vi "权值计算.vi"(0 "当前棋盘状态":i32[][](array[numeric])) -> (3 "权值最大的三个位置":dbl[][](array[numeric]), 4 "当前棋盘状态":i32[][](array[numeric]), 8 "行":sgl, 10 "列":i16, 13 "黑子最大权值":sgl, 14 "白子最大权值":sgl format="%#_0f", 15 "白子权值大于黑子？":bool)   [LabVIEW 2018]
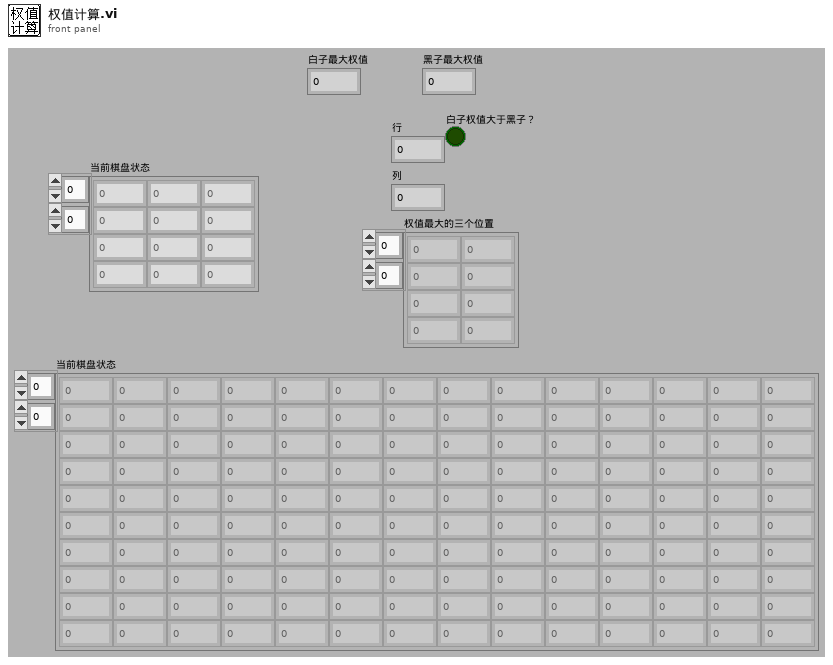
[diagram p1: front panel]
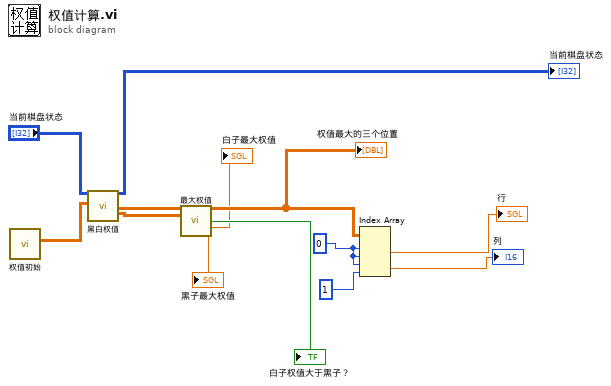
[diagram p0: block diagram]
diagram:
  w7 = 0 ("index (row)")
  n1 = call "权值初始.vi"() -> ("初始棋盘权值"=w12:sgl[][])  [unwired: 11 in]
  n2 = call "黑白权值.vi"("输入棋盘状态"="当前棋盘状态", "初始棋盘权值"=w12) -> ("输出棋盘状态"=→"当前棋盘状态":i32[][], "白子棋盘总权值"=w10:sgl[][], "黑子棋盘总权值"=w9:sgl[][])  [unwired: 15 in]
  n3 = call "最大权值.vi"("白子棋盘权值"=w10, "黑子棋盘权值"=w9) -> ("权值最大的前三个位置"=w8:dbl[][], "白子权值勤大于黑子？"=→"白子权值大于黑子？":bool, "白子最大权值"=→"白子最大权值":sgl, "黑子最大权值"=→"黑子最大权值":sgl)  [unwired: 10 in]
  "权值最大的三个位置" <- w8
  n4 = Index Array(array=w8, index (row) #1=w7, index (col) #1=w7, index (row) #2=w7, index (col) #2=1 ("index (row)")) -> (element #1=→"行":dbl, element #2=→"列":dbl)
